vi "Stop Live.vi"(0 "Camera reference in":refnum<k24>, 5 "Error In":errorcluster) -> (14 "Camera reference out":refnum<k24>, 19 "Error Out":errorcluster)   [LabVIEW 2017]
uses:
  C:/Program Files/National Instruments/LabVIEW 2017/instr.lib/IDS/ueye.NET/uEyeDotNet.dll
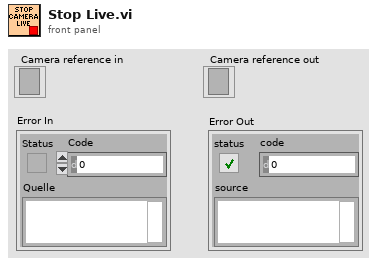
[diagram p1: front panel]
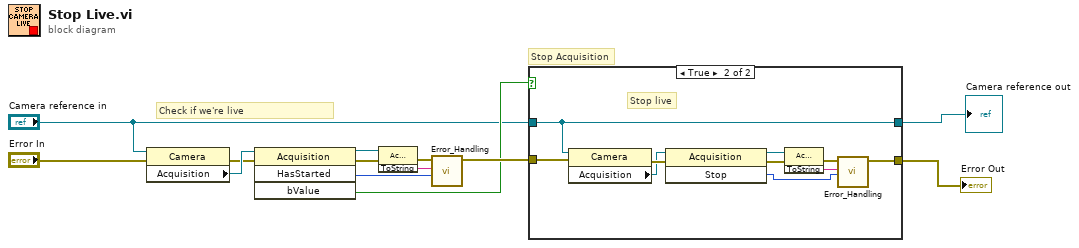
[diagram p0: block diagram]
diagram:
  # "Check if we're live"
  # "Stop Acquisition"
  n1 = property class="Camera"(reference="Camera reference in", error in="Error In") -> (error out=w5:errorcluster, "Acquisition"=w6:refnum<k24>)  [unwired: 1 out]
  n2 = invoke class="Acquisition" method="HasStarted"(reference=w6, error in=w5) -> (reference out=w10:refnum<k24>, error out=w11:errorcluster, "HasStarted"=w12:i32, "bValue"=w7:bool)  [unwired: 2 in]
  n3 = invoke class="Acquisition" method="ToString"(reference=w10, error in=w11) -> (error out=w8:errorcluster, "ToString"=w9:string)  [unwired: 1 in, 1 out]
  n4 = call <instrlib>:"Error_Handling.vi"("Error Code"=w12, "Error String"=w9, "Error In"=w8) -> ("Error Out"=w13:errorcluster)  [unwired: 8 in]
  n5 = case shown="True" w7 {
    tunnel: [w14 w16] -> w4
    tunnel: w13 -> [w14 w23]
    tunnel: "Camera reference in" -> [w15 w22]
    tunnel: [w15 w22] -> w3
    frame False {
      # "We're already stopped!"
    }
    frame True {
      # "Stop live"
      n6 = property class="Camera"(reference=w22, error in=w23) -> (error out=w25:errorcluster, "Acquisition"=w24:refnum<k24>)  [unwired: 1 out]
      n7 = invoke class="Acquisition" method="Stop"(reference=w24, error in=w25) -> (reference out=w19:refnum<k24>, error out=w18:errorcluster, "Stop"=w17:i32)  [unwired: 1 in]
      n8 = invoke class="Acquisition" method="ToString"(reference=w19, error in=w18) -> (error out=w21:errorcluster, "ToString"=w20:string)  [unwired: 1 in, 1 out]
      n9 = call <instrlib>:"Error_Handling.vi"("Error Code"=w17, "Error String"=w20, "Error In"=w21) -> ("Error Out"=w16:errorcluster)  [unwired: 8 in]
    }
  }
  "Error Out" <- w4
  "Camera reference out" <- w3
